vi "testUserStopsServersAandB.vi"(8 "error in":errorcluster) -> (0 "error out":errorcluster)   [LabVIEW 2018]
uses:
  src/TcpServer/TcpServer.lvclass
  <vilib>/addons/_JKI Toolkits/Caraya/classes/Assert/Assert Not Error.vi
  <vilib>/addons/_JKI Toolkits/Caraya/classes/Test/Test.lvclass
  <vilib>/addons/_JKI Toolkits/Caraya/classes/Assert/Assert.lvclass
panel:
  out "Run Server B error":errorcluster
  out "Run Server A error":errorcluster
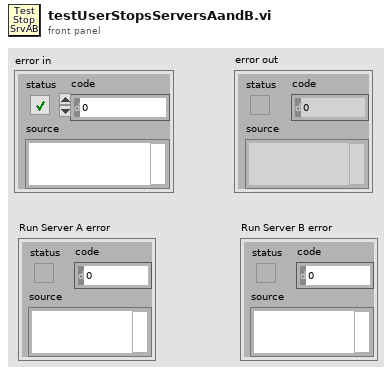
[diagram p1: front panel]
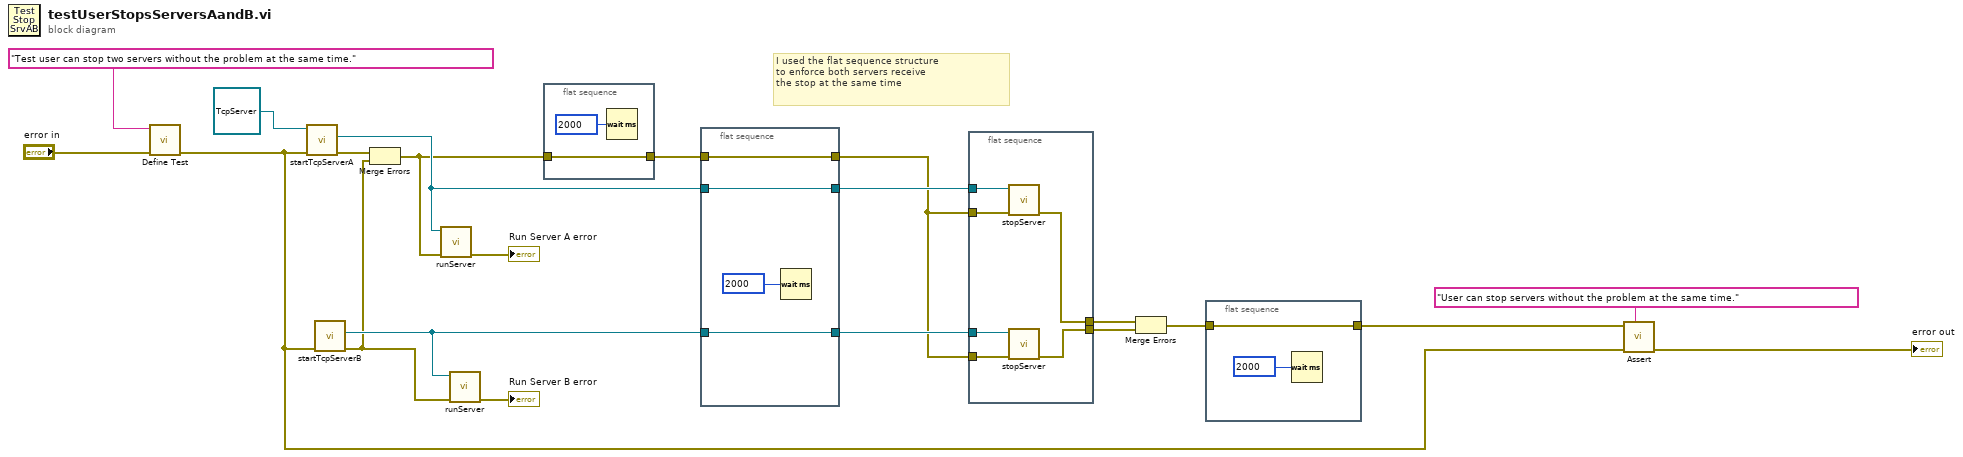
[diagram p0: block diagram]
diagram:
  # "I used the flat sequence structure\nto enforce both servers receive\nthe stop at the same time"
  n1 = call <vilib>:"Define Test.vi"("error in (no error)"="error in", "Label (VI Title)"="Test user can stop two servers without the problem at the same time.") -> ("error out"=w4:errorcluster)  [unwired: 9 in]
  n2 = call "startTcpServerA.vi"("error in (no error)"=w4, "TcpServer.lvclass"=refnum<class "TcpServer.lvclass"> refnum) -> ("error out"=w19:errorcluster, "TcpServer out"=w13:refnum<class "TcpServer.lvclass">)  [unwired: 7 in, 1 out]
  n3 = call "startTcpServerB.vi"("error in (no error)"=w4) -> ("error out"=w2:errorcluster, "TcpServer out"=w11:refnum<class "TcpServer.lvclass">)  [unwired: 8 in, 1 out]
  n4 = Merge Errors(w19, w2) -> (w3:errorcluster)
  n5 = call "runServer.vi"("error in (no error)"=w3, "TcpServer in"=w13) -> ("error out (no error)"=→"Run Server A error":errorcluster)  [unwired: 8 in, 1 out]
  n6 = call "runServer.vi"("error in (no error)"=w2, "TcpServer in"=w11) -> ("error out (no error)"=→"Run Server B error":errorcluster)  [unwired: 8 in, 1 out]
  n7 = flat-sequence {
    tunnel: w3 -> [w22]
    tunnel: [w22] -> w10
    frame #0 {
      n8 = Wait (ms)(milliseconds to wait=u32 2000) -> ()  [unwired: 1 out]
    }
  }
  n9 = flat-sequence {
    tunnel: [w26] -> w14
    tunnel: w13 -> [w26]
    tunnel: [w25] -> w12
    tunnel: w11 -> [w25]
    tunnel: w10 -> [w24]
    tunnel: [w24] -> w9
    frame #0 {
      n10 = Wait (ms)(milliseconds to wait=u32 2000) -> ()  [unwired: 1 out]
    }
  }
  n11 = flat-sequence {
    tunnel: [w33] -> w18
    tunnel: [w32] -> w17
    tunnel: w14 -> [w31]
    tunnel: w12 -> [w30]
    tunnel: w9 -> [w29]
    tunnel: w9 -> [w28]
    frame #0 {
      n12 = call "stopServer.vi"("error in (no error)"=w29, "tcpServer in"=w31) -> ("error out"=w33:errorcluster)  [unwired: 8 in, 1 out]
      n13 = call "stopServer.vi"("error in (no error)"=w28, "tcpServer in"=w30) -> ("error out"=w32:errorcluster)  [unwired: 8 in, 1 out]
    }
  }
  n14 = Merge Errors(w18, w17) -> (w16:errorcluster)
  n15 = flat-sequence {
    tunnel: w16 -> [w35]
    tunnel: [w35] -> w5
    frame #0 {
      n16 = Wait (ms)(milliseconds to wait=u32 2000) -> ()  [unwired: 1 out]
    }
  }
  n17 = call-poly <vilib>:"Assert.vi"("Label"="User can stop servers without the problem at the same time.", "error in (no error)"=w4, "Not Error?"=w5) -> ("error out"=→"error out":errorcluster)  [unwired: 8 in]
